vi "Scan Nodes.vi"(8 "error in (no error)":errorcluster, 9 "timeout_ms":u64=2000, 10 "Query Expression":string="*", 11 "Zenoh in":refnum<class "Zenoh.lvclass">) -> (0 "error out":errorcluster, 3 "Nodes":string[](array[string]))   [LabVIEW 2021, in "Zenoh.lvclass"]
doc: "Scan for Zenoh nodes on the network."
uses:
  Zenoh.lvclass
  Zenoh.lvclass/Zenoh.ctl
  SubVIs/Get Zenoh Path.vi
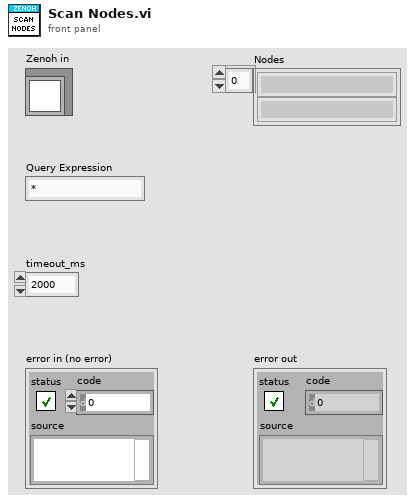
[diagram p1: front panel]
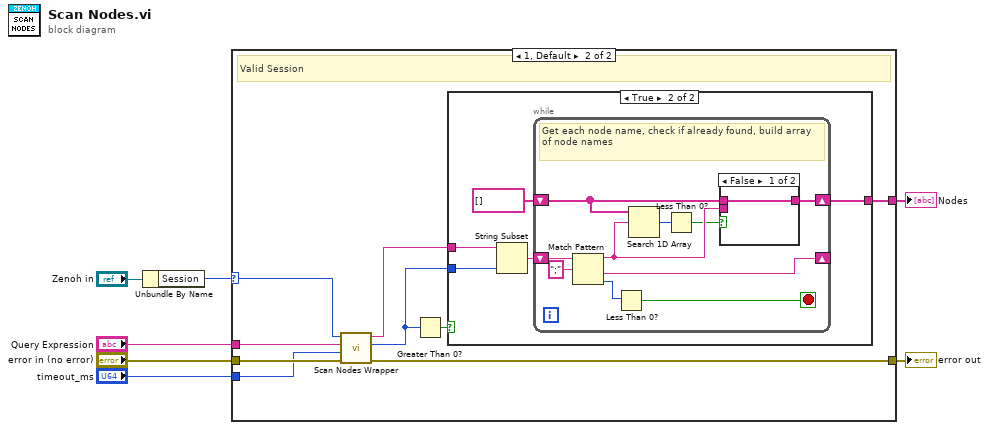
[diagram p0: block diagram]
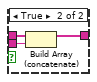
[diagram p4: hidden frame]
diagram:
  n1 = Unbundle By Name("Zenoh in") -> ("Session"=w5:u64)
  n2 = case shown="1, Default" w5 {
    selector: w5 -> [_ w13]
    tunnel: "Query Expression" -> [_ w15]
    tunnel: "error in (no error)" -> [w8 w17]
    tunnel: [w8 w16] -> w4
    tunnel: "timeout_ms" -> [_ w14]
    tunnel: [_ w9] -> w1
    frame 0 {
      # "Invalid session"
    }
    frame 1, Default {
      # "Valid Session"
      n3 = call "Scan Nodes Wrapper.vi"("error in (no error)"=w17, "timeout_ms"=w14, "Key Filter"=w15, "Reader Handle"=w13) -> ("error out"=w16:errorcluster, "Length"=w11:i32, "buffer_out"=w12:string)  [unwired: 5 in]
      n4 = Greater Than 0?(x=w11) -> (x > 0?=w10:bool)
      n5 = case shown="True" w10 {
        tunnel: w11 -> [_ w22]
        tunnel: w12 -> [_ w21]
        tunnel: [_ w19] -> w9
        frame False {
        }
        frame True {
          n6 = String Subset(string=w21, length (rest)=w22) -> (substring=w20:string)  [unwired: 1 in]
          n7 = while {
            shift-right: [w28] -> _
            shift-left: w20 -> [w32]
            shift-right: [w27] -> w19
            shift-left: string[] [] -> [w25]
            stop <- w29 stop-if-true
            # "Get each node name, check if already found, build array of node names"
            n8 = Match Pattern(string=w32, regular expression=";") -> (before substring=w24:string, after substring=w28:string, offset past match=w30:i32)  [unwired: 1 in, 1 out]
            n9 = Less Than 0?(x=w30) -> (x < 0?=w29:bool)
            n10 = Search 1D Array(1D array=w25, element=w24) -> (index of element=w26:i32)  [unwired: 1 in]
            n11 = Less Than 0?(x=w26) -> (x < 0?=w23:bool)
            n12 = case shown="False" w23 {
              tunnel: [w33 w36] -> w27
              tunnel: w25 -> [w33 w35]
              tunnel: w24 -> [_ w34]
              frame False {
              }
              frame True {
                n13 = Build Array (concatenate)(w35, w34) -> (w36:string[])
              }
            }
          }
        }
      }
    }
  }
  "error out" <- w4
  "Nodes" <- w1
